vi "MessageBase.getFieldSpecByName.vi"(8 "error in (no error)":errorcluster, 10 "Field.Name":string="Canceled Quantity", 11 "MessageBase in":refnum<class "MessageBase.lvclass">) -> (0 "error out":errorcluster, 2 "FIeldSpec":T1, 3 "MessageBase out":refnum<class "MessageBase.lvclass">)   [LabVIEW 2020, in "MessageBase.lvclass"]
uses:
  MessageBase.lvclass
  FieldSpec.ctl
  MessageBase.lvclass/MessageBase.ctl
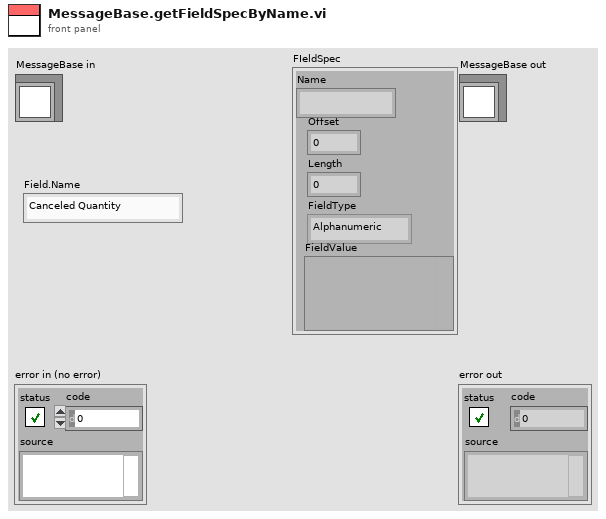
[diagram p1: front panel]
types:
  T1 = typedef "FieldSpec.ctl" = cluster{"Name":string, "Offset":i32, "Length":i32, "FieldType":enum16{"Alphanumeric", "Binary", "BinaryLongPrice", "BinaryShortPrice", "BitField", "PrintableAscii", "Value"}, "FieldValue":variant}
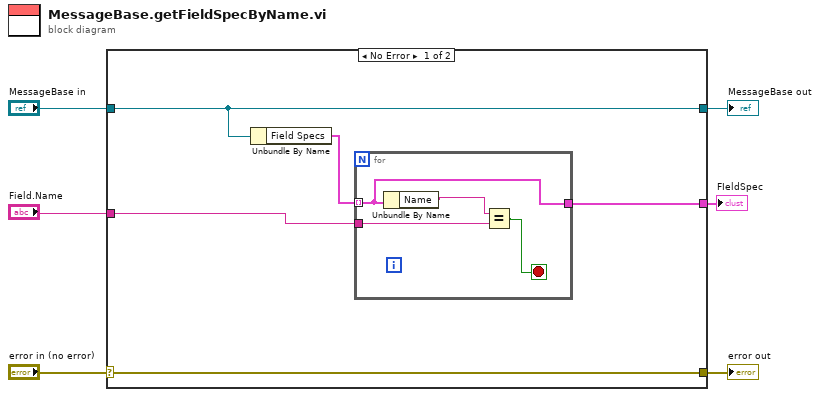
[diagram p0: block diagram]
diagram:
  n1 = case shown="No Error" "error in (no error)" {
    selector: "error in (no error)" -> [w11 w17]
    tunnel: [w11 w17] -> w5
    tunnel: [w8 w16] -> w3
    tunnel: "MessageBase in" -> [w8 w16]
    tunnel: "Field.Name" -> [w9 _]
    tunnel: [w7 _] -> w1
    frame No Error {
      n2 = Unbundle By Name(w8) -> ("Field Specs"=w10:T1[])
      n3 = for {
        tunnel: w10 -> [w12] mode=indexing
        tunnel: w9 -> [w15]
        tunnel: [w12] -> w7
        stop <- w14 stop-if-true
        n4 = Unbundle By Name(w12) -> ("Name"=w13:string)
        n5 = Equal?(x=w13, y=w15) -> (x = y?=w14:bool)
      }
    }
    frame Error {
    }
  }
  "error out" <- w5
  "MessageBase out" <- w3
  "FIeldSpec" <- w1
